vi "Janis_RealtimeRvT_1Channel_LR700.vi"() -> ()   [LabVIEW 2014]
uses:
  <vilib>/Utility/file.llb/Write To Spreadsheet File (DBL).vi
panel:
  out "TimeStamp":dbl format="%#_13g"
  out "T2":dbl
  out "T1":dbl
  out "X1":dbl
  in  "Tab Control":enum32{"Set Up"}(tab)
  in  "LR700\nAddress":i16
  in  "LKS Temp Controller":refnum<visa-resource-name>
  in  "SampleName":string
  in  "Sample \nThermometer":enum16{"T1", "T2"}(ring)
  out "XY Graph 6":cluster{dbl, dbl}[](graph) caption="Temp Channel A"
  out "XY Graph 5":cluster{dbl, dbl}[](graph) caption="Temp Channel B"
  out "XY Graph 4":cluster{dbl, dbl}[](graph) caption="SRS1"
  out "Data is being stored here":string
  # "RealTime Data"
  # "Thermometry"
  # "INSTRUMENT ADDRESSES"
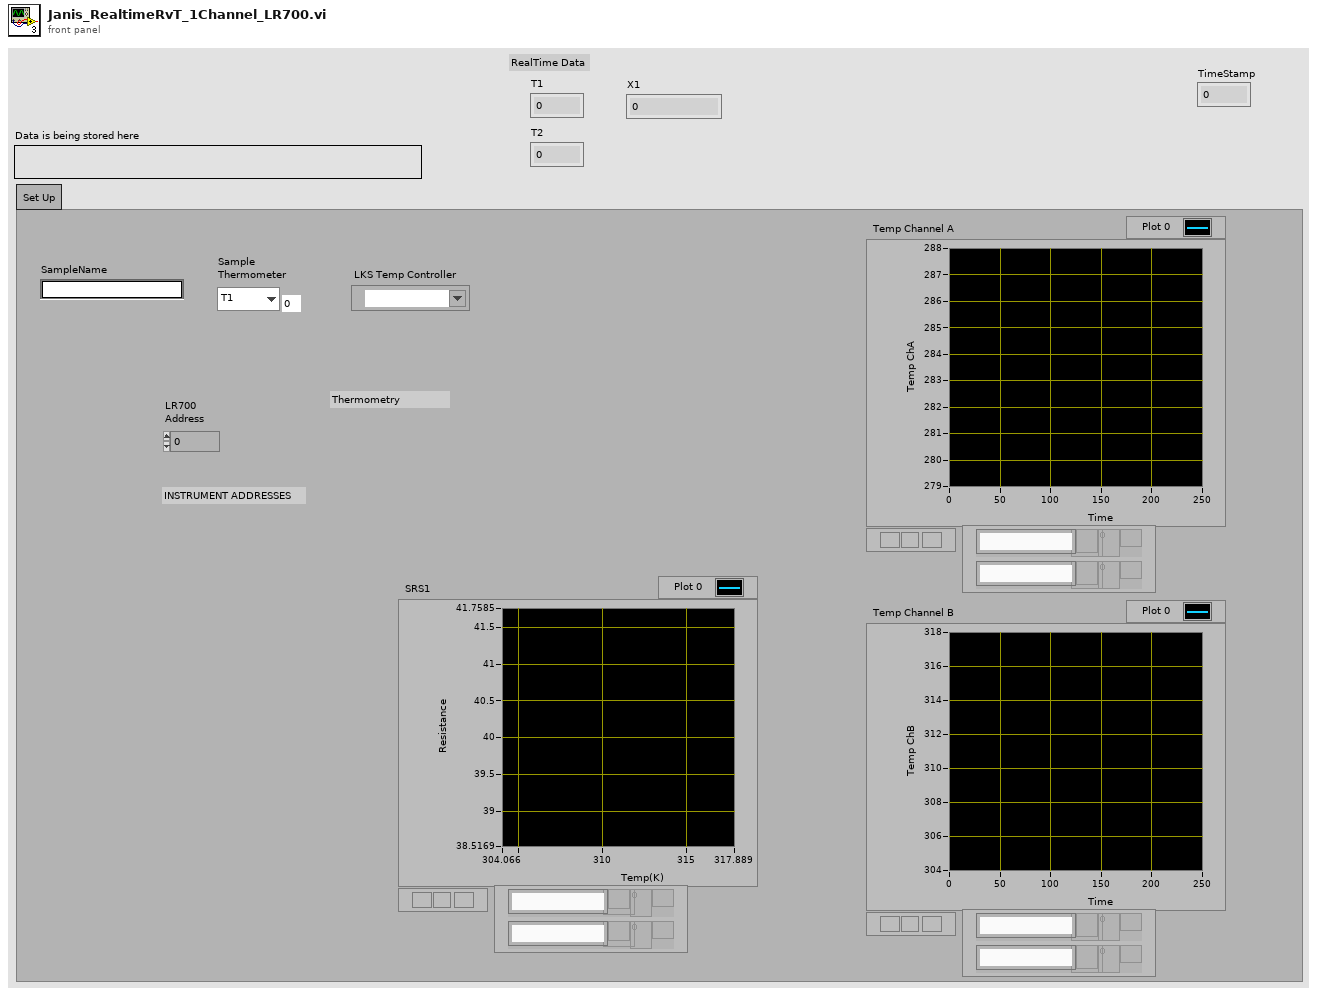
[diagram p1: front panel]
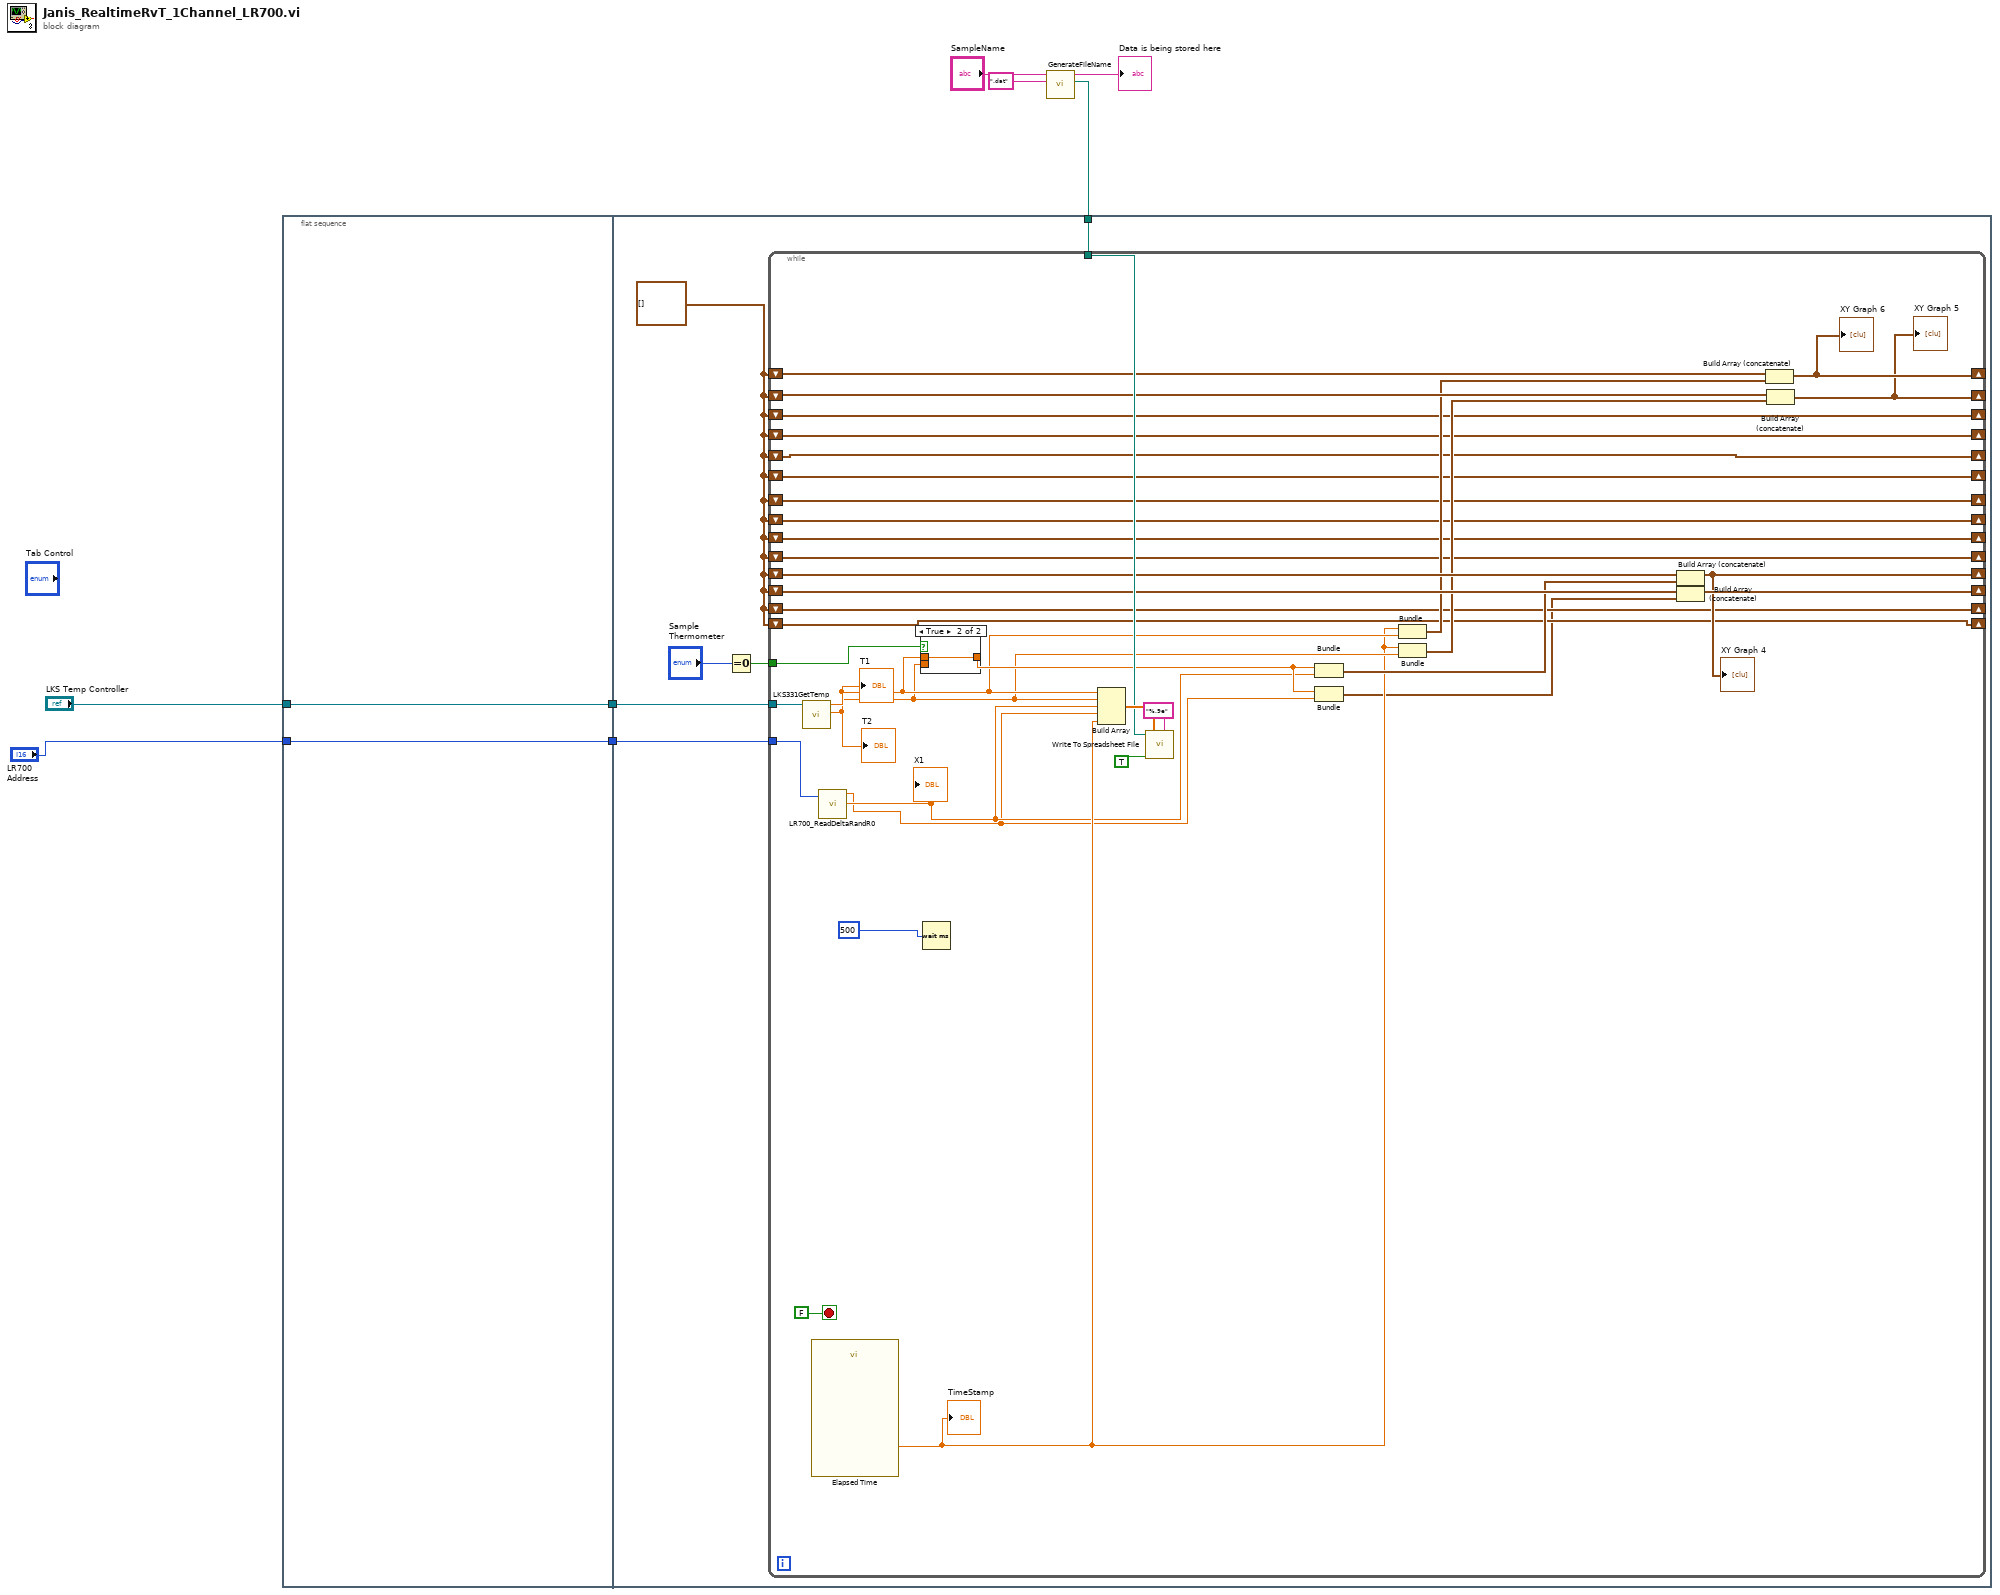
[diagram p0: block diagram]
diagram:
  n1 = flat-sequence {
    tunnel: "LR700\nAddress" -> [w9]
    tunnel: "LKS Temp Controller" -> [w10]
    tunnel: [w10] -> w4
    tunnel: [w9] -> w3
    tunnel: w4 -> [w16]
    tunnel: w3 -> [w15]
    tunnel: w2 -> [w14]
    frame #0 {
    }
    frame #1 {
      w11 = cluster{"T1":dbl, "Elapsed Time (s)":dbl}[] []
      n2 = Equal To 0?(x="Sample \nThermometer") -> (x = 0?=w13:bool)
      n3 = while {
        tunnel: w16 -> [w52]
        tunnel: w15 -> [w20]
        tunnel: w14 -> [w48]
        tunnel: w13 -> [w47]
        shift-right: [w23] -> _
        shift-left: w11 -> [w23]
        shift-right: [w22] -> _
        shift-left: w11 -> [w22]
        shift-right: [w43] -> _
        shift-left: w11 -> [w45]
        shift-right: [w32] -> _
        shift-left: w11 -> [w46]
        shift-right: [w24] -> _
        shift-left: w11 -> [w24]
        shift-right: [w26] -> _
        shift-left: w11 -> [w26]
        shift-right: [w27] -> _
        shift-left: w11 -> [w27]
        shift-right: [w25] -> _
        shift-left: w11 -> [w25]
        shift-right: [w31] -> _
        shift-left: w11 -> [w31]
        shift-right: [w30] -> _
        shift-left: w11 -> [w30]
        shift-right: [w29] -> _
        shift-left: w11 -> [w29]
        shift-right: [w28] -> _
        shift-left: w11 -> [w28]
        shift-right: [w35] -> _
        shift-left: w11 -> [w41]
        shift-right: [w34] -> _
        shift-left: w11 -> [w40]
        stop <- FALSE stop-if-true
        n4 = call "LKS331GetTemp.vi"("LKS Temp Controller"=w52) -> ("T2"=w38:dbl, "T1"=w39:dbl)  [unwired: 8 in, 1 out]
        "T1" <- w39
        "T2" <- w38
        n5 = call "Elapsed Time"() -> ("Elapsed Time (s)"=w33:dbl)  [unwired: 12 in, 7 out]
        "TimeStamp" <- w33
        n6 = call "LR700_ReadDeltaRandR0.vi"("LR700\nAddress"=w20) -> ("R0"=w19:dbl, "DeltaR"=w18:dbl)  [unwired: 8 in, 1 out]
        "X1" <- w19
        n7 = case shown="True" w47 {
          tunnel: w39 -> [_ w55]
          tunnel: w38 -> [w54 _]
          tunnel: [w54 w55] -> w42
          frame False {
          }
          frame True {
          }
        }
        n8 = Wait (ms)(milliseconds to wait=500) -> ()  [unwired: 1 out]
        n9 = Build Array(w39, w38, w19, w18, w33) -> (w51:dbl[])
        n10 = call-poly <vilib>:"Write To Spreadsheet File.vi"("format (%.3f)"="%.9e", "append to file? (new file:F)"=TRUE, "1D data"=w51, "file path (dialog if empty)"=w48) -> ()  [unwired: 4 in, 1 out]
        n11 = Bundle("T1"=w42, "R0"=w19) -> (w44:cluster{"T1":dbl, "R0":dbl})  [unwired: 1 in]
        n12 = Bundle("T1"=w42, "DeltaR"=w18) -> (w21:cluster{"T1":dbl, "DeltaR":dbl})  [unwired: 1 in]
        n13 = Bundle("Elapsed Time (s)"=w33, "T1"=w39) -> (w36:cluster{"Elapsed Time (s)":dbl, "T1":dbl})  [unwired: 1 in]
        n14 = Bundle("Elapsed Time (s)"=w33, "T2"=w38) -> (w37:cluster{"Elapsed Time (s)":dbl, "T2":dbl})  [unwired: 1 in]
        n15 = Build Array (concatenate)(w46, w44) -> (w32:cluster{"T1":dbl, "R0":dbl}[])
        "XY Graph 4" <- w32
        n16 = Build Array (concatenate)(w45, w21) -> (w43:cluster{"T1":dbl, "DeltaR":dbl}[])
        n17 = Build Array (concatenate)(w41, w36) -> (w35:cluster{"Elapsed Time (s)":dbl, "T1":dbl}[])
        "XY Graph 6" <- w35
        n18 = Build Array (concatenate)(w40, w37) -> (w34:cluster{"Elapsed Time (s)":dbl, "T2":dbl}[])
        "XY Graph 5" <- w34
      }
    }
  }
  n19 = call "GenerateFileName.vi"("FileExtension"=".dat", "SampleName"="SampleName") -> ("FilePathOut"=w2:path, "FolderNameString"=→"Data is being stored here":string)  [unwired: 3 in, 1 out]
